vi "Ass3.vi"() -> ()   [LabVIEW 2018]
uses:
  Control 4.ctl
  <vilib>/measure/NI_MABase.lvlib
panel:
  out "DEMm2(t)":dynamicdata(graph)
  out "m2(t)":dynamicdata(graph)
  out "DEMm1(t)":dynamicdata(graph)
  out "m1(t)":dynamicdata(graph)
  in  "phase 2":dbl format="%.2p"
  in  "phase":T1 format="%.2p"
  in  "seed 2":i32=-1
  in  "amplitude 3":dbl=1.0 format="%0.2p"
  in  "frequency 2":dbl=10.0 format="%0.2p"
  in  "seed":i32=-1
  in  "amplitude 2":dbl=1.0 format="%.2p"
  in  "sampling info":cluster{"Fs":dbl, "#s":dbl}={"Fs"=1000.0, "#s"=1000.0} {"Fs" format="%.2p"}
  in  "amplitude":dbl=1.0 format="%0.2p"
  in  "frequency":dbl=10.0 format="%0.2p"
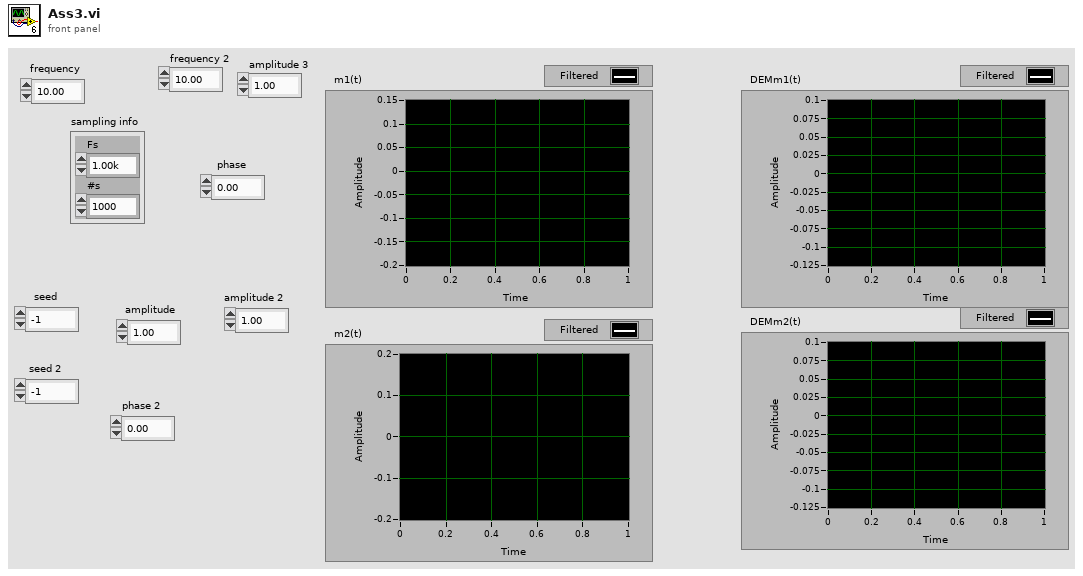
[diagram p1: front panel]
types:
  T1 = typedef "Control 4.ctl" = dbl
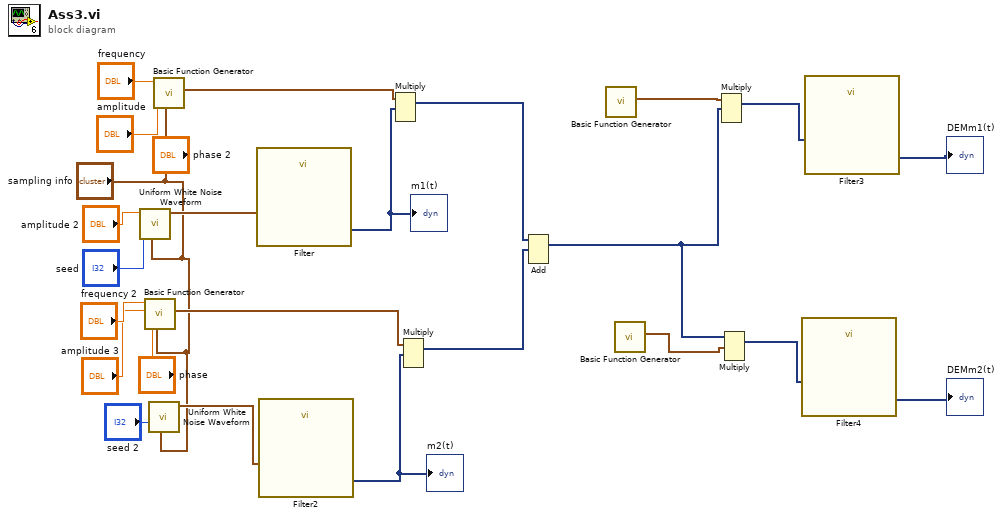
[diagram p0: block diagram]
diagram:
  n1 = call <vilib>:"Uniform White Noise Waveform.vi"("sampling info"="sampling info", "seed"="seed", "amplitude"="amplitude 2") -> ("signal out"=w25:waveform(dbl))  [unwired: 7 in, 1 out]
  n2 = call <vilib>:"Basic Function Generator.vi"("sampling info"="sampling info", "phase"="phase", "amplitude"="amplitude 3", "frequency"="frequency 2") -> ("signal out"=w22:waveform(dbl))  [unwired: 5 in, 2 out]
  n3 = call <vilib>:"Uniform White Noise Waveform.vi"("sampling info"="sampling info", "seed"="seed 2") -> ("signal out"=w24:waveform(dbl))  [unwired: 8 in, 1 out]
  n4 = call <vilib>:"Basic Function Generator.vi"("sampling info"="sampling info", "phase"="phase 2", "amplitude"="amplitude", "frequency"="frequency") -> ("signal out"=w23:waveform(dbl))  [unwired: 5 in, 2 out]
  n5 = call "Filter"("Signal"=w25) -> ("Filtered Signal"=w2:dynamicdata)  [unwired: 9 in, 1 out]
  "m1(t)" <- w2
  n6 = call "Filter2"("Signal"=w24) -> ("Filtered Signal"=w1:dynamicdata)  [unwired: 9 in, 1 out]
  "m2(t)" <- w1
  n7 = Multiply(1:w2, 2:w23) -> (0:w13:dynamicdata)  [unwired: 1 in, 1 out]
  n8 = Multiply(1:w1, 2:w22) -> (0:w12:dynamicdata)  [unwired: 1 in, 1 out]
  n9 = Add(1:w12, 2:w13) -> (0:w8:dynamicdata)  [unwired: 1 in, 1 out]
  n10 = call <vilib>:"Basic Function Generator.vi"() -> ("signal out"=w9:waveform(dbl))  [unwired: 9 in, 2 out]
  n11 = call <vilib>:"Basic Function Generator.vi"() -> ("signal out"=w7:waveform(dbl))  [unwired: 9 in, 2 out]
  n12 = Multiply(1:w8, 2:w9) -> (0:w6:dynamicdata)  [unwired: 1 in, 1 out]
  n13 = Multiply(1:w7, 2:w8) -> (0:w5:dynamicdata)  [unwired: 1 in, 1 out]
  n14 = call "Filter4"("Signal"=w5) -> ("Filtered Signal"=→"DEMm2(t)":dynamicdata)  [unwired: 9 in, 1 out]
  n15 = call "Filter3"("Signal"=w6) -> ("Filtered Signal"=→"DEMm1(t)":dynamicdata)  [unwired: 9 in, 1 out]
